vi "ai kalman step.vi"(9 "AI look-ahead":i16, 10 "val in":i32, 11 "Kalman PV state in":T1) -> (2 "estimate":i16, 3 "kalman pv state out":T1)   [LabVIEW 2010]
uses:
  kalman pv state.ctl
  <vilib>/rvi/FXPMathLib/FxpMul/XNode/nifxpmath_Multiplier.xnode
  <vilib>/rvi/FXPMathLib/FxpMul/subVIs/nifxpmath_Mul_SimConfig.ctl
  <vilib>/fxp/LVFixedPointQuantizationPolicyTypeDef.ctl
  <vilib>/fxp/LVFixedPointOverflowPolicyTypeDef.ctl
  <vilib>/rvi/FXPMathLib/FxpMul/simVIs/DllFxpMulTemp_sub.vi
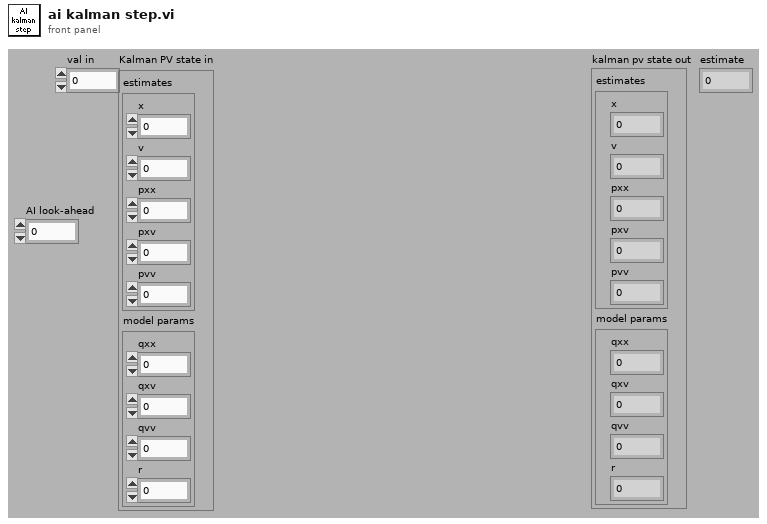
[diagram p1: front panel]
types:
  T1 = typedef "kalman pv state.ctl" = cluster{"estimates":cluster{"x":fxp<+/-,18,16>, "v":fxp<+/-,18,16>, "pxx":u16, "pxv":u16, "pvv":u16}, "model params":cluster{"qxx":u16, "qxv":u16, "qvv":u16, "r":u16}}
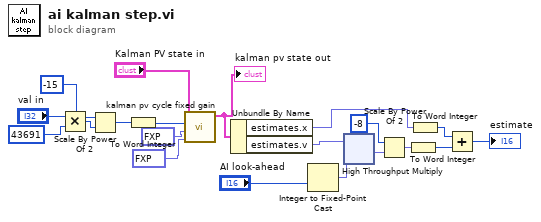
[diagram p0: block diagram]
diagram:
  n1 = Multiply(x="val in", y=43691) -> (x*y=w6:i32)
  n2 = Scale By Power Of 2(n=-15, x=w6) -> (x*2^n=w7:i32)
  n3 = To Word Integer(number=w7) -> (16bit integer=w8:i16)
  n4 = call "kalman pv cycle fixed gain.vi"("v gain"=fxp<+,16,0> 0.136993408203125, "x gain"=fxp<+,16,0> 0.4766998291015625, "position measurement"=w8, "Kalman PV state"="Kalman PV state in") -> ("kalman pv state out"=w9:T1)  [unwired: 7 in]
  "kalman pv state out" <- w9
  n5 = Unbundle By Name(w9) -> ("estimates.x"=w3:fxp<+/-,18,16>, "estimates.v"=w19:fxp<+/-,18,16>)
  n6 = Integer to Fixed-Point Cast(integer="AI look-ahead") -> (fixed-point=w18:fxp<+/-,16,16>)  [unwired: 1 in]
  n7 = xnode "High Throughput Multiply"("x"=w19, "y"=w18) -> ("x*y"=w17:fxp<+/-,24,24>)
  n8 = Scale By Power Of 2(n=-8, x=w17) -> (x*2^n=w16:fxp<+/-,24,24>)
  n9 = To Word Integer(number=w16) -> (16bit integer=w15:i16)
  n10 = To Word Integer(number=w3) -> (16bit integer=w14:i16)
  n11 = Add(x=w14, y=w15) -> (x+y=→"estimate":i16)
